vi "Git_UserInfo.vi"(4 "Your Password (not necessary)":string, 6 "Your User Name (not necessary)":string, 8 "error in (no error)":errorcluster, 11 "Repo User Name":string) -> (0 "error out":errorcluster, 1 "Not Found?":bool, 2 "body":string, 3 "headers":string)   [LabVIEW 2012]
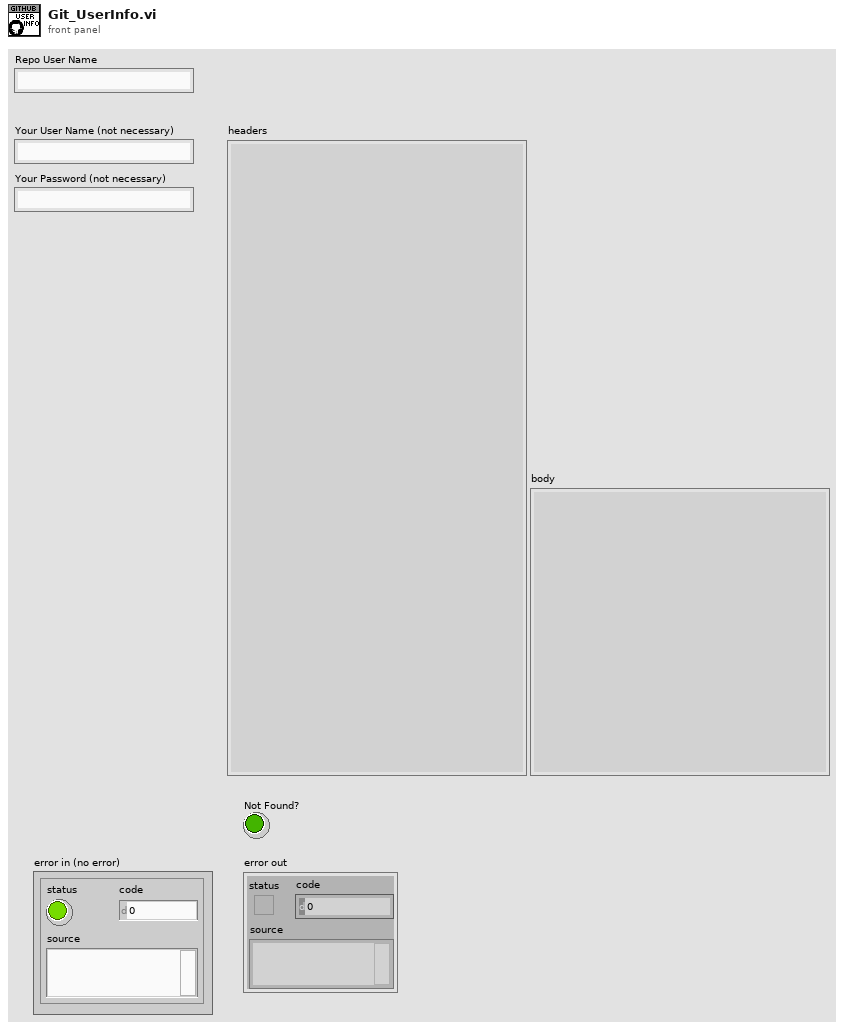
[diagram p1: front panel]
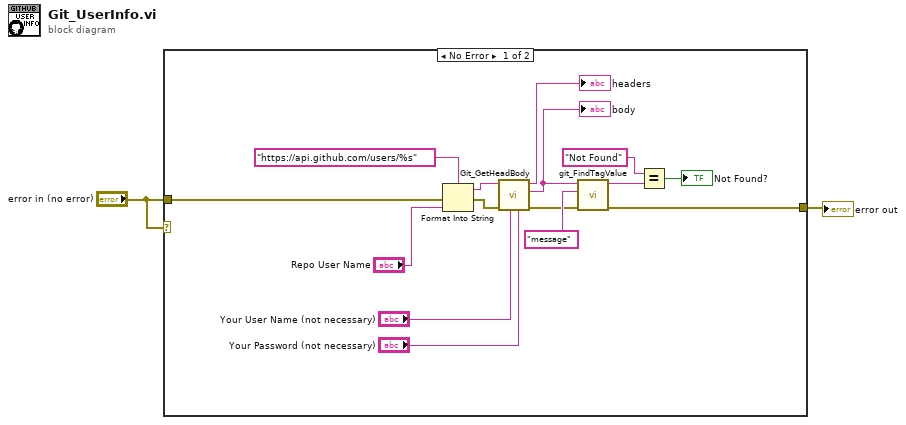
[diagram p0: block diagram]
diagram:
  n1 = case shown="No Error" "error in (no error)" {
    tunnel: [w17 w18] -> w2
    tunnel: "error in (no error)" -> [w10 w18]
    frame No Error {
      n2 = Format Into String(format string="https://api.github.com/users/%s", error in=w10, "Repo User Name") -> (resulting string=w9:string, error out=w11:errorcluster)  [unwired: 1 in]
      n3 = call "Git_GetHeadBody.vi"("Your Password (not necessary)"="Your Password (not necessary)", "Your User Name (not necessary)"="Your User Name (not necessary)", "error in (no error)"=w11, "Address"=w9) -> ("error out"=w5:errorcluster, "body"=w12:string, "headers"=→"headers":string)  [unwired: 5 in]
      "body" <- w12
      n4 = call "git_FindTagValue.vi"("Error In"=w5, "Tag Name"="message", "Text"=w12) -> ("Error Out"=w17:errorcluster, "Value"=w14:string)  [unwired: 6 in, 1 out]
      n5 = Equal?(x="Not Found", y=w14) -> (x = y?=→"Not Found?":bool)
    }
    frame Error {
    }
  }
  "error out" <- w2
